vi "process.vi"(8 "error in (no error)":errorcluster, 11 "Subscription in":refnum<class "Subscription.lvclass">) -> ()   [LabVIEW 2013, in "MQTT Server.lvlib" / "Subscription.lvclass"]
uses:
  Subscription.lvclass
  <vilib>/LabVIEW Open Source Project/MQTT Control Packets/Control Packets/ControlPacket/QualityOfService -- enum.ctl
  Subscription.lvclass/Subscription.ctl
  TopicFilter/TopicFilter.lvclass/TopicFilter.ctl
  <vilib>/LabVIEW Open Source Project/MQTT Control Packets/Control Packets/ControlPacket/ControlPacket.lvclass/ControlPacket.ctl
  <vilib>/LabVIEW Open Source Project/MQTT Control Packets/Control Packets/Ack/Ack.lvclass
  <vilib>/LabVIEW Open Source Project/MQTT Control Packets/Control Packets/PUBLISH/PUBLISH.lvclass
  <vilib>/LabVIEW Open Source Project/MQTT Control Packets/Control Packets/ControlPacket/ControlPacket.lvclass
panel:
  out "QoS":T1
  out "Topic Filter":string
  out "Numeric":i32
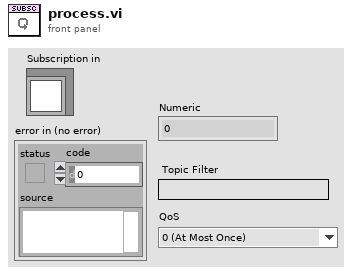
[diagram p1: front panel]
types:
  T1 = typedef "MQTT_Control_Packets.lvlib/ControlPacket.lvclass/QualityOfService -- enum.ctl" = enum16{"0 (At Most Once)", "1 (At Least Once)", "2 (Exactly Once)"}
  T2 = typedef "MQTT Server.lvlib/Subscription.lvclass/Stored Packet -- cluster.ctl" = cluster{"Packet Identifier":u16, "ControlPacket":refnum<class "ControlPacket.lvclass">, "last attempt":timestamp}
  T3 = typedef "MQTT_Control_Packets.lvlib/ControlPacket.lvclass/Control Packet Type -- enum.ctl" = enum16{"Reserved", "CONNECT", "CONNACK", "PUBLISH", "PUBACK", "PUBREC", "PUBREL", "PUBCOMP", "SUBSCRIBE", "SUBACK", "UNSUBSCRIBE", "UNSUBACK", "PINGREQ", "PINGRESP", "DISCONNECT", "AUTH"}
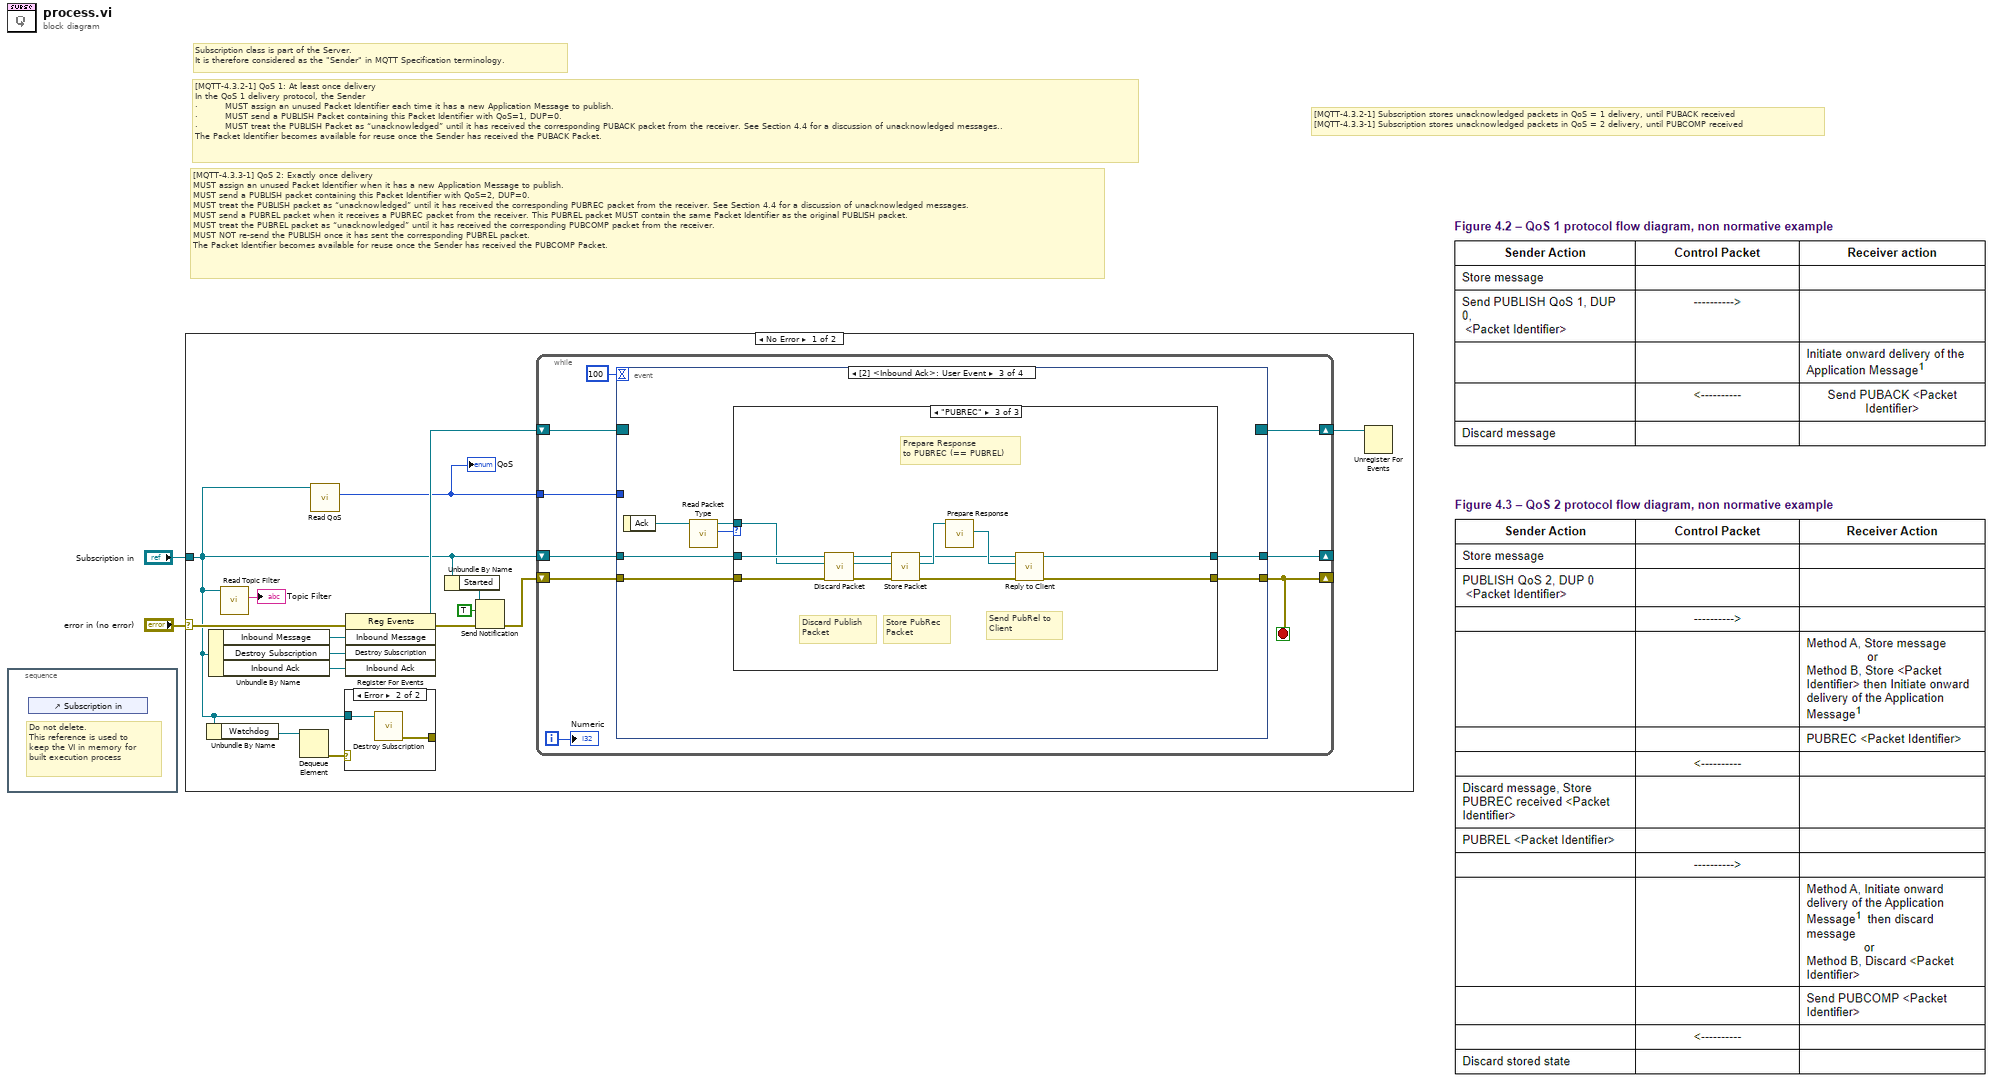
[diagram p0: block diagram]
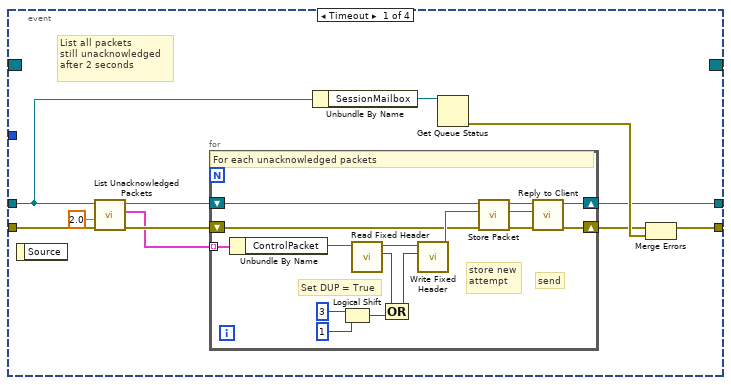
[diagram p3: hidden frame]
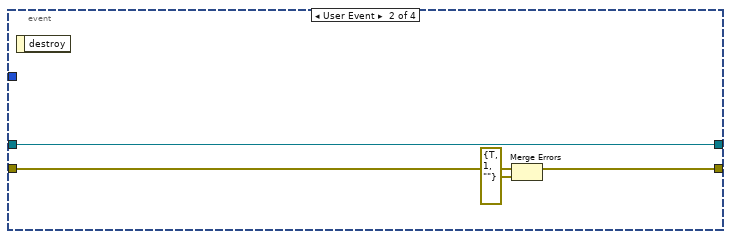
[diagram p4: hidden frame]
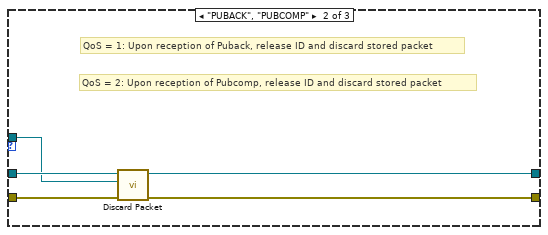
[diagram p6: hidden frame]
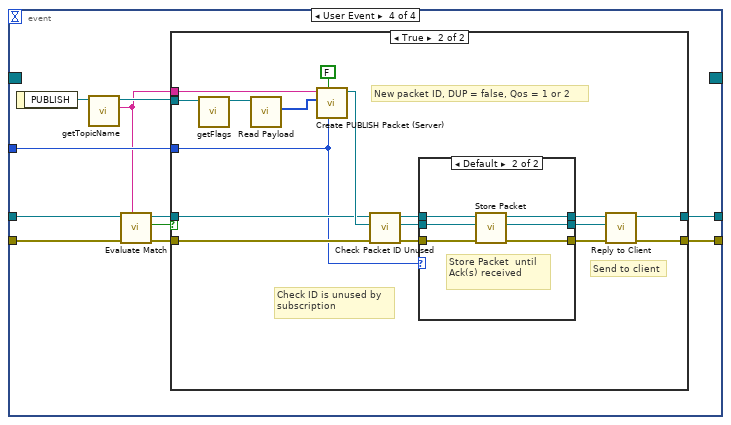
[diagram p7: hidden frame]
diagram:
  # "[MQTT-4.3.2-1] Subscription stores unacknowledged packets in QoS = 1 delivery, until PUBACK received\n[MQTT-4.3.3-1] Subscription stores unacknowledged packets in QoS = 2 delivery, until PUBCOMP received"
  # "[MQTT-4.3.3-1] QoS 2: Exactly once delivery\nMUST assign an unused Packet Identifier when it has a new Application Message to publish.\nMUST send a PUBLISH packet containing this Packet Identifier with QoS=2, DUP=0.\nMUST treat the PUBLISH packet as “unacknowledged” until it has received the corresponding PUBREC packet from the receiver. See Section 4.4 for a discussion of unacknowledged messages.\nMUST send a PUBREL packet when it receives a PUBREC packet from the receiver. This PUBREL packet MUST contain the same Packet Identifier as the original PUBLISH packet.\nMUST treat the PUBREL packet as “unacknowledged” until it has received the corresponding PUBCOMP packet from the receiver.\nMUST NOT re-send the PUBLISH once it has sent the corresponding PUBREL packet.\nThe Packet Identifier becomes available for reuse once the Sender has received the PUBCOMP Packet."
  # "[MQTT-4.3.2-1] QoS 1: At least once delivery\nIn the QoS 1 delivery protocol, the Sender\n·         MUST assign an unused Packet Identifier each time it has a new Application Message to publish.\n·         MUST send a PUBLISH Packet containing this Packet Identifier with QoS=1, DUP=0.\n·         MUST treat the PUBLISH Packet as “unacknowledged” until it has received the corresponding PUBACK packet from the receiver. See Section 4.4 for a discussion of unacknowledged messages..\nThe Packet Identifier becomes available for reuse once the Sender has received the PUBACK Packet."
  # "Subscription class is part of the Server.\nIt is therefore considered as the \"Sender\" in MQTT Specification terminology."
  n1 = stacked-sequence {
    frame #0 {
      # "Do not delete.\nThis reference is used to keep the VI in memory for built execution process"
      n2 = control-ref of="Subscription in"() -> ()  [unwired: 1 out]
    }
  }
  n3 = case shown="No Error" "error in (no error)" {
    selector: "error in (no error)" -> [w15 _]
    tunnel: "Subscription in" -> [w4 _]
    frame No Error {
      n4 = Unbundle By Name(w4) -> ("Watchdog"=w10:refnum<queue>)
      n5 = Unbundle By Name(w4) -> ("Inbound Message"=w8:refnum<user-event>, "Destroy Subscription"=w7:refnum<user-event>, "Inbound Ack"=w5:refnum<user-event>)
      n6 = call "Read Topic Filter.vi"("Subscription in"=w4) -> ("Topic Filter"=→"Topic Filter":string)  [unwired: 7 in, 3 out]
      n7 = Dequeue Element(queue=w10) -> (error out=w9:errorcluster)  [unwired: 2 in, 3 out]
      n8 = call "Read QoS.vi"("Subscription in"=w4) -> ("QoS"=w3:T1)  [unwired: 8 in, 2 out]
      "QoS" <- w3
      n9 = case shown="Error" w9 {
        tunnel: w4 -> [_ w19]
        tunnel: [_ w18] -> _
        frame No Error {
        }
        frame Error {
          n10 = call "Destroy Subscription.vi"("Subscription in"=w19) -> ("error out"=w18:errorcluster)  [unwired: 9 in, 1 out]
        }
      }
      n11 = register-events(error in=w15, w8, w7, w5) -> (reference out=w13:refnum<event-registration>, error out=w14:errorcluster)  [unwired: 1 in]
      n12 = Unbundle By Name(w4) -> ("Started"=w6:refnum<notifier>)
      n13 = Send Notification(notification=TRUE, notifier=w6, error in (no error)=w14) -> (error out=w16:errorcluster)  [unwired: 1 out]
      n14 = while {
        shift-right: [w24] -> _
        shift-left: w16 -> [w20]
        shift-right: [w26] -> w12
        shift-left: w13 -> [w27]
        shift-right: [w22] -> _
        shift-left: w4 -> [w25]
        tunnel: w3 -> [w21]
        i -> [w23]
        stop <- w24 stop-if-true
        n15 = event shown="[2] <Inbound Ack>: User Event" {
          selector: w27 -> [_ _ _ _]
          dyn-events: [_ _ _ _] -> w26
          timeout: 100 -> [_ _ _ _]
          tunnel: w25 -> [w36 w58 w64 w89]
          tunnel: [w37 w59 w60 w96] -> w24
          tunnel: [w32 w58 w61 w91] -> w22
          tunnel: w21 -> [_ _ _ w87]
          tunnel: w20 -> [w35 w56 w63 w88]
          event Timeout {
            # "List all packets\nstill unacknowledged\nafter 2 seconds"
            n16 = event-data() -> ()  [unwired: 1 in, 1 out]
            n17 = call "List Unacknowledged Packets.vi"("error in (no error)"=w35, "filter (0s: list all)"=2.0, "Subscription in"=w36) -> ("error out"=w31:errorcluster, "Unacknowledged"=w29:T2[], "Subscription out"=w33:refnum<class "Subscription.lvclass">)  [unwired: 6 in]
            n18 = for {
              shift-right: [w47] -> w32
              shift-left: w33 -> [w45]
              shift-right: [w46] -> w30
              shift-left: w31 -> [w41]
              tunnel: w29 -> [w55] mode=indexing
              # "send"
              # "store new\nattempt"
              # "Set DUP = True"
              # "For each unacknowledged packets"
              n19 = Unbundle By Name(w55) -> ("ControlPacket"=w50:refnum<class "ControlPacket.lvclass">)
              n20 = Logical Shift(y=i16 3, x=u8 1) -> (x << y=w51:u8)
              n21 = call <vilib>:"Read Fixed Header.vi"("ControlPacket in"=w50) -> ("Fixed Header"=w49:u8, "ControlPacket out"=w54:refnum<class "ControlPacket.lvclass">)  [unwired: 9 in]
              n22 = Compound Arithmetic op=OR(w49, w51) -> (w48:u8)
              n23 = call <vilib>:"Write Fixed Header.vi"("Fixed Header"=w48, "ControlPacket in"=w54) -> ("ControlPacket out"=w43:refnum<class "ControlPacket.lvclass">)  [unwired: 9 in]
              n24 = call "Store Packet.vi"("error in (no error)"=w41, "ControlPacket"=w43, "Subscription in"=w45) -> ("error out"=w40:errorcluster, "ControlPacket dup"=w42:refnum<class "ControlPacket.lvclass">, "Subscription out"=w44:refnum<class "Subscription.lvclass">)  [unwired: 6 in]
              n25 = call "Reply to Client.vi"("error in (no error)"=w40, "ControlPacket"=w42, "Subscription in"=w44) -> ("error out"=w46:errorcluster, "Subscription out"=w47:refnum<class "Subscription.lvclass">)  [unwired: 7 in]
            }
            n26 = Unbundle By Name(w36) -> ("SessionMailbox"=w39:refnum<queue>)
            n27 = Get Queue Status(queue=w39) -> (error out=w38:errorcluster)  [unwired: 2 in, 7 out]
            n28 = Merge Errors(w30, w38) -> (w37:errorcluster)
          }
          event User Event {
            n29 = event-data() -> ()  [unwired: 1 in, 1 out]
            n30 = Merge Errors(w56, errorcluster {"status"=TRUE, "code"=1, "source"=""} ("error in")) -> (w59:errorcluster)
          }
          event User Event {
            n31 = event-data() -> ("Ack"=w66:refnum<class "Ack.lvclass">)  [unwired: 1 in]
            n32 = call <vilib>:"Read Packet Type.vi"("ControlPacket in"=w66) -> ("Control Packet Type"=w65:T3, "ControlPacket out"=w62:refnum<class "Ack.lvclass">)  [unwired: 9 in]
            n33 = case shown="\"PUBREC\"" w65 {
              tunnel: w64 -> [w68 w73 w85]
              tunnel: w63 -> [w67 w71 w83]
              tunnel: w62 -> [_ w72 w84]
              tunnel: [w68 w70 w76] -> w61
              tunnel: [w67 w69 w74] -> w60
              frame Default {
                # "Already discarded packets.\nDuplicates ==> ignore"
              }
              frame "PUBACK", "PUBCOMP" {
                # "QoS = 2: Upon reception of Pubcomp, release ID and discard stored packet"
                # "QoS = 1: Upon reception of Puback, release ID and discard stored packet"
                n34 = call "Discard Packet.vi"("error in (no error)"=w71, "Ack"=w72, "Subscription in"=w73) -> ("error out"=w69:errorcluster, "Subscription out"=w70:refnum<class "Subscription.lvclass">)  [unwired: 5 in, 2 out]
              }
              frame "PUBREC" {
                # "Prepare Response\nto PUBREC (== PUBREL)"
                # "Send PubRel to\nClient"
                # "Store PubRec\nPacket"
                # "Discard Publish\nPacket"
                n35 = call "Discard Packet.vi"("error in (no error)"=w83, "Ack"=w84, "Subscription in"=w85) -> ("error out"=w80:errorcluster, "Ack dup"=w81:refnum<class "Ack.lvclass">, "Subscription out"=w82:refnum<class "Subscription.lvclass">)  [unwired: 5 in, 1 out]
                n36 = call "Store Packet.vi"("error in (no error)"=w80, "ControlPacket"=w81, "Subscription in"=w82) -> ("error out"=w75:errorcluster, "ControlPacket dup"=w79:refnum<class "Ack.lvclass">, "Subscription out"=w77:refnum<class "Subscription.lvclass">)  [unwired: 6 in]
                n37 = call-dynamic "Prepare Response.vi"("ControlPacket in"=w79) -> ("ControlPacket response"=w78:refnum<class "ControlPacket.lvclass">)  [unwired: 7 in, 3 out]
                n38 = call "Reply to Client.vi"("error in (no error)"=w75, "ControlPacket"=w78, "Subscription in"=w77) -> ("error out"=w74:errorcluster, "Subscription out"=w76:refnum<class "Subscription.lvclass">)  [unwired: 7 in]
              }
            }
          }
          event User Event {
            n39 = event-data() -> ("PUBLISH"=w90:refnum<class "PUBLISH.lvclass">)  [unwired: 1 in]
            n40 = call <vilib>:"getTopicName.vi"("PUBLISH in"=w90) -> ("Topic"=w86:string, "PUBLISH out"=w95:refnum<class "PUBLISH.lvclass">)  [unwired: 8 in, 1 out]
            n41 = call "Evaluate Match.vi"("Topic"=w86, "error in (no error)"=w88, "Subscription in"=w89) -> ("error out"=w92:errorcluster, "Matched"=w94:bool, "Subscription out"=w93:refnum<class "Subscription.lvclass">)  [unwired: 5 in, 1 out]
            n42 = case shown="True" w94 {
              tunnel: [w98 w115] -> w96
              tunnel: w92 -> [w98 w107]
              tunnel: w93 -> [w97 w103]
              tunnel: w95 -> [_ w101]
              tunnel: [w97 w114] -> w91
              tunnel: w86 -> [_ w113]
              tunnel: w87 -> [_ w99]
              frame False {
                # "Not a match for subscription"
              }
              frame True {
                # "New packet ID, DUP = false, Qos = 1 or 2"
                # "Send to client"
                # "Check ID is unused by\nsubscription"
                n43 = call-dynamic "getFlags.vi"("PUBLISH in"=w101) -> ("PUBLISH out"=w100:refnum<class "PUBLISH.lvclass">)  [unwired: 7 in, 3 out]
                n44 = call <vilib>:"Read Payload.vi"("ControlPacket in"=w100) -> ("Payload"=w111:u8[])  [unwired: 9 in, 1 out]
                n45 = call <vilib>:"Create PUBLISH Packet (Server).vi"("QoS"=w99, "DUP (Re-delivery attempt)"=FALSE, "Payload"=w111, "Topic Name"=w113) -> ("PUBLISH"=w105:refnum<class "PUBLISH.lvclass">)  [unwired: 4 in, 3 out]
                n46 = call "Check Packet ID Unused.vi"("error in (no error)"=w107, "PUBLISH"=w105, "Subscription in"=w103) -> ("error out"=w106:errorcluster, "PUBLISH out"=w104:refnum<class "PUBLISH.lvclass">, "Subscription out"=w102:refnum<class "Subscription.lvclass">)  [unwired: 6 in]
                n47 = case shown="Default" w99 {
                  tunnel: w102 -> [w118 w124]
                  tunnel: [w118 w123] -> w110
                  tunnel: [w117 w120] -> w109
                  tunnel: w106 -> [w117 w121]
                  tunnel: w104 -> [w116 w122]
                  tunnel: [w116 w119] -> w108
                  frame "0 (At Most Once)" {
                  }
                  frame Default {
                    # "Store Packet  until Ack(s) received"
                    n48 = call "Store Packet.vi"("error in (no error)"=w121, "ControlPacket"=w122, "Subscription in"=w124) -> ("error out"=w120:errorcluster, "ControlPacket dup"=w119:refnum<class "PUBLISH.lvclass">, "Subscription out"=w123:refnum<class "Subscription.lvclass">)  [unwired: 6 in]
                  }
                }
                n49 = call "Reply to Client.vi"("error in (no error)"=w109, "ControlPacket"=w108, "Subscription in"=w110) -> ("error out"=w115:errorcluster, "Subscription out"=w114:refnum<class "Subscription.lvclass">)  [unwired: 7 in]
              }
            }
          }
        }
        "Numeric" <- w23
      }
      n50 = Unregister For Events(event registration refnum=w12) -> ()  [unwired: 1 in, 1 out]
    }
    frame Error {
    }
  }
